vi "Position Out of Bounds Test.vi"(5 "VI reference":refnum<vi>, 7 "Center Bounds":T3, 8 "error in":errorcluster, 11 "Editor Position in":refnum<class "Editor Position.lvclass">) -> (0 "error out":errorcluster, 3 "Editor Position out":refnum<class "Editor Position.lvclass">)   [LabVIEW 2020, in "Editor Position.lvclass"]
doc: "Tests how the Set Editor Position reacts to a position that is outside of any monitor bounds."
uses:
  Editor Position.lvclass
  Editor Position.lvclass/Editor Position.ctl
  vi.lib/LabVIEW Icon API/lv_icon/lv_icon.lvlib
  <vilib>/Utility/miscctls.llb/LVRectTypeDef.ctl
  1c0a1d1d-4178-4595-873d-4a9a1072f670.vi
  <vilib>/Utility/miscctls.llb/LVAllMonitorsDisplayTypeDef.ctl
panel:
  out "Display:All Monitors":T1
  out "Tested Positions":T2(array[cluster])
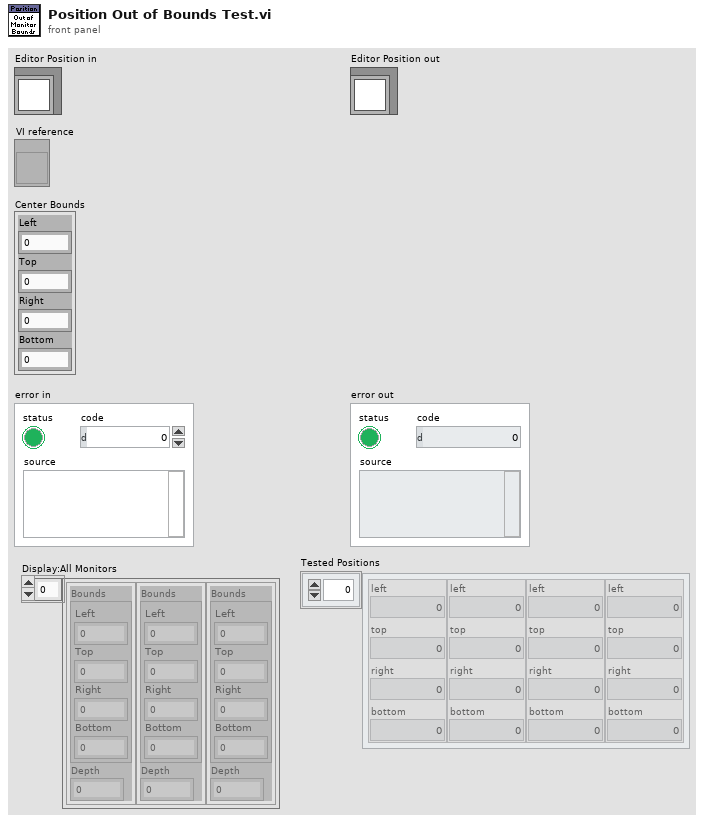
[diagram p1: front panel]
types:
  T1 = typedef "LVAllMonitorsDisplayTypeDef.ctl" = cluster{"Bounds":cluster{"Left":i16, "Top":i16, "Right":i16, "Bottom":i16}, "Depth":i16}[]
  T2 = cluster{"left":i16, "top":i16, "right":i16, "bottom":i16}[]
  T3 = typedef "LVRectTypeDef.ctl" = cluster{"Left":i16, "Top":i16, "Right":i16, "Bottom":i16}
  T4 = cluster{"left":i16, "top":i16, "right":i16, "bottom":i16}
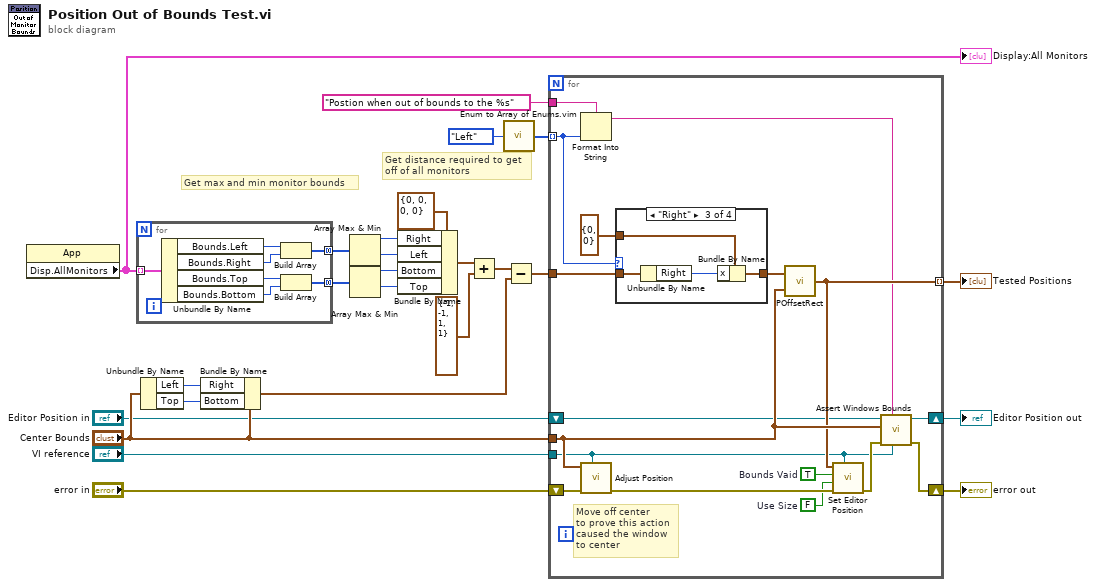
[diagram p0: block diagram]
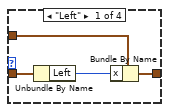
[diagram p2: hidden frame]
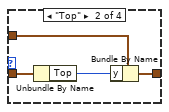
[diagram p3: hidden frame]
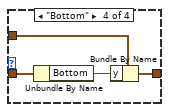
[diagram p4: hidden frame]
diagram:
  # "Get distance required to get\noff of all monitors"
  # "Get max and min monitor bounds"
  n1 = property class="App"() -> ("Disp.AllMonitors"=w6:T1)  [unwired: 2 in, 2 out]
  "Display:All Monitors" <- w6
  n2 = for {
    tunnel: w6 -> [w32] mode=indexing
    tunnel: [w27] -> w22 mode=concatenating
    tunnel: [w26] -> w21 mode=concatenating
    n3 = Unbundle By Name(w32) -> ("Bounds.Left"=w31:i16, "Bounds.Right"=w30:i16, "Bounds.Top"=w29:i16, "Bounds.Bottom"=w28:i16)
    n4 = Build Array(w31, w30) -> (w27:i16[])
    n5 = Build Array(w29, w28) -> (w26:i16[])
  }
  n6 = Unbundle By Name("Center Bounds") -> ("Left"=w3:i16, "Top"=w2:i16)
  n7 = Bundle By Name(cluster="Center Bounds", "Right"=w3, "Bottom"=w2) -> (w5:T3)
  n8 = Array Max & Min(array=w22) -> (max value=w19:i16, min value=w18:i16)  [unwired: 2 out]
  n9 = Array Max & Min(array=w21) -> (max value=w17:i16, min value=w16:i16)  [unwired: 2 out]
  n10 = Bundle By Name(cluster=T3 {"Left"=0, "Top"=0, "Right"=0, "Bottom"=0} ("Center Bounds"), "Right"=w19, "Left"=w18, "Bottom"=w17, "Top"=w16) -> (w15:T3)
  n11 = Add(x=w15, y=T3 {"Left"=-1, "Top"=-1, "Right"=1, "Bottom"=1}) -> (x+y=w14:T3)
  n12 = call "Enum to Array of Enums.vim"("enum"=enum8{"Left", "Top", "Right", "Bottom"}."Left") -> ("array of enums"=w10:enum8{"Left", "Top", "Right", "Bottom"}[])
  n13 = Subtract(x=w14, y=w5) -> (x-y=w8:T3)
  n14 = for {
    tunnel: "VI reference" -> [w33]
    tunnel: "Center Bounds" -> [w45]
    shift-right: [w35] -> w12
    shift-left: "Editor Position in" -> [w36]
    shift-right: [w46] -> w24
    shift-left: "error in" -> [w49]
    tunnel: w10 -> [w42] mode=indexing
    tunnel: "Postion when out of bounds to the %s" ("format string") -> [w43]
    tunnel: w8 -> [w41]
    tunnel: [w44] -> w7 mode=indexing
    w38 = FALSE  # Use Size
    w39 = TRUE  # Bounds Vaid
    # "Move off center\nto prove this action\ncaused the window\nto center"
    n15 = Format Into String(format string=w43, w42) -> (resulting string=w34:string)  [unwired: 2 in, 1 out]
    n16 = call "Adjust Position.vi"("VI in"=w33, "error in"=w49, "Current Position"=w45) -> ("error out"=w48:errorcluster)  [unwired: 7 in, 1 out]
    n17 = case shown="\"Right\"" w42 {
      tunnel: w41 -> [w52 w56 w60 w64]
      tunnel: cluster{"x":i16, "y":i16} {"x"=0, "y"=0} ("point") -> [w53 w57 w61 w65]
      tunnel: [w50 w54 w58 w62] -> w37
      frame "Left" {
        n18 = Unbundle By Name(w52) -> ("Left"=w51:i16)
        n19 = Bundle By Name(cluster=w53, "x"=w51) -> (w50:cluster{"x":i16, "y":i16})
      }
      frame "Top" {
        n20 = Unbundle By Name(w56) -> ("Top"=w55:i16)
        n21 = Bundle By Name(cluster=w57, "y"=w55) -> (w54:cluster{"x":i16, "y":i16})
      }
      frame "Right" {
        n22 = Unbundle By Name(w60) -> ("Right"=w59:i16)
        n23 = Bundle By Name(cluster=w61, "x"=w59) -> (w58:cluster{"x":i16, "y":i16})
      }
      frame "Bottom" {
        n24 = Unbundle By Name(w64) -> ("Bottom"=w63:i16)
        n25 = Bundle By Name(cluster=w65, "y"=w63) -> (w62:cluster{"x":i16, "y":i16})
      }
    }
    n26 = call <vilib>:"POffsetRect.vi"("rect"=w45, "point"=w37) -> ("offset rect"=w44:T4)
    n27 = call "Set Editor Position.vi"("IE VI Ref"=w33, "error in"=w48, "Use Size"=w38, "Bounds Vaid"=w39, "Window Bounds"=w44) -> ("error out"=w47:errorcluster)  [unwired: 6 in]
    n28 = call "Assert Windows Bounds.vi"("VI reference"=w33, "Test Description"=w34, "error in"=w47, "Expected Position"=w45, "Editor Position in"=w36) -> ("error out"=w46:errorcluster, "Editor Position out"=w35:refnum<class "Editor Position.lvclass">)  [unwired: 5 in]
  }
  "error out" <- w24
  "Editor Position out" <- w12
  "Tested Positions" <- w7
